vi "calculate image sharpness.vi"(8 "error in (no error)":errorcluster, 9 "Sharpness measure":T1, 11 "Autofocus in":refnum<class "Autofocus.lvclass">) -> (0 "error out":errorcluster, 2 "sharpness out":dbl, 3 "Autofocus out":refnum<class "Autofocus.lvclass">)   [LabVIEW 2012, in "Autofocus.lvclass"]
uses:
  Autofocus.lvclass
  Sharpness Measure.ctl
  Autofocus.lvclass/Autofocus.ctl
  search direction.ctl
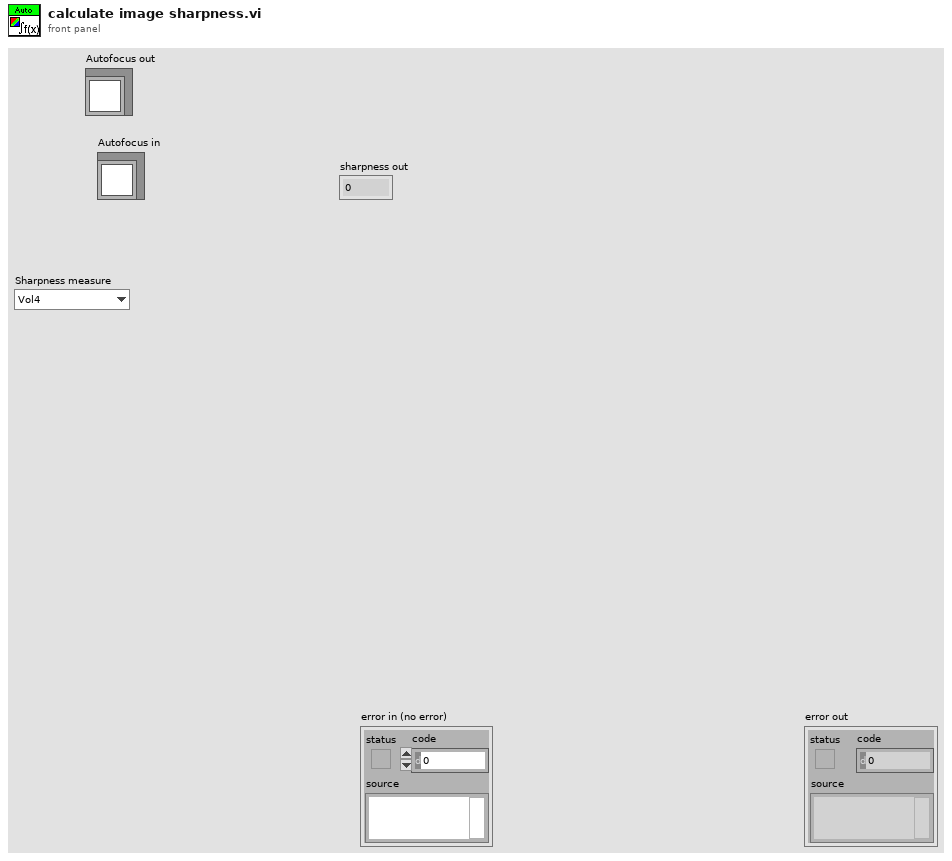
[diagram p1: front panel]
types:
  T1 = typedef "Autofocus.lvclass/Sharpness Measure.ctl" = enum16{"Vol4", "Gradient Square"}
  T2 = typedef "Autofocus.lvclass/search direction.ctl" = enum16{"going uphill", "going downhill", "idle"}
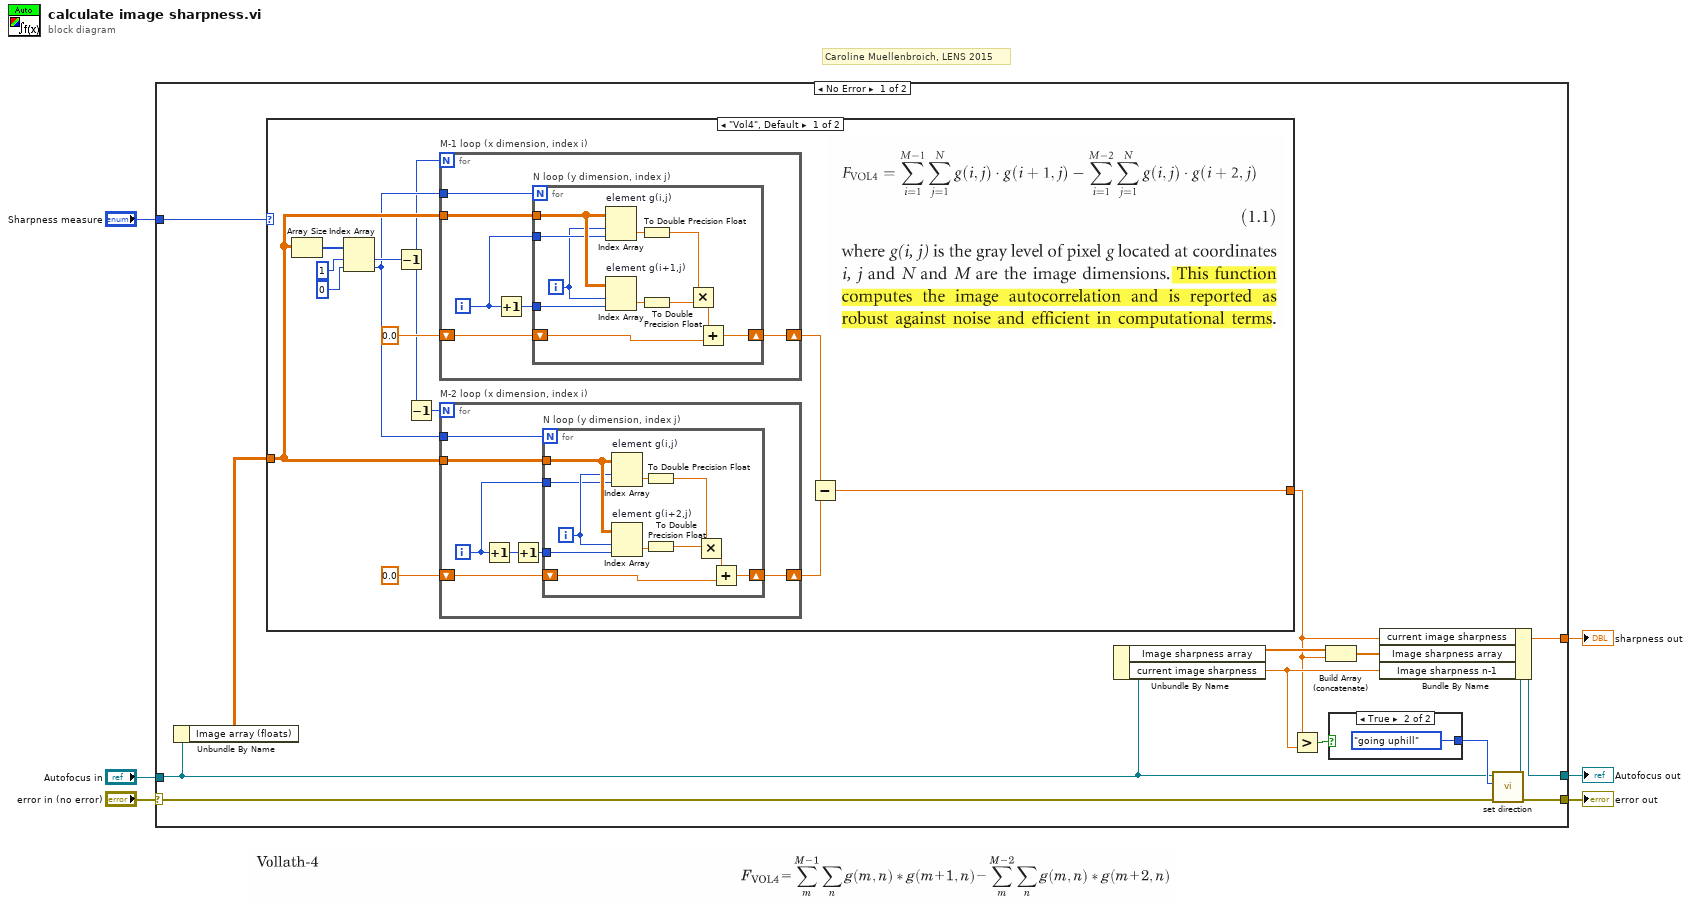
[diagram p0: block diagram]
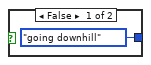
[diagram p2: hidden frame]
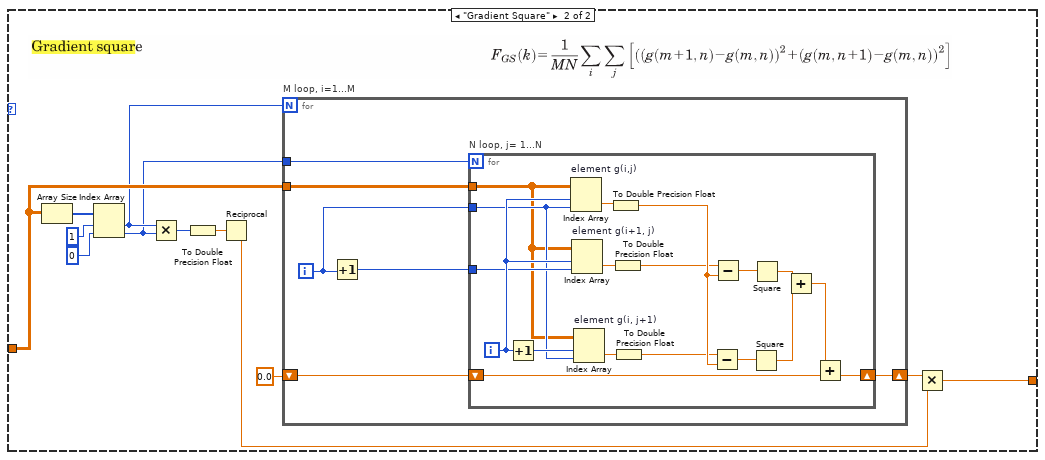
[diagram p3: hidden frame]
diagram:
  # "Caroline Muellenbroich, LENS 2015"
  n1 = case shown="No Error" "error in (no error)" {
    selector: "error in (no error)" -> [w10 w107]
    tunnel: [w15 w107] -> w5
    tunnel: [w19 w106] -> w3
    tunnel: "Autofocus in" -> [w8 w106]
    tunnel: [w11 _] -> w2
    tunnel: "Sharpness measure" -> [w18 _]
    frame No Error {
      n2 = Unbundle By Name(w8) -> ("Image array (floats)"=w7:dbl[][])
      n3 = case shown="\"Vol4\", Default" w18 {
        tunnel: w7 -> [w29 w78]
        tunnel: [w23 w73] -> w11
        frame "Vol4", Default {
          n4 = Array Size(array=w29) -> (size(s)=w34:i32[])
          n5 = Index Array(array=w34, index #1=1 ("index"), index #2=0 ("index")) -> (element #1=w30:i32, element #2=w28:i32)
          n6 = Decrement(x=w30) -> (x-1=w22:i32)
          n7 = Decrement(x=w22) -> (x-1=w31:i32)
          n8 = for "M-1 loop (x dimension, index i)" {
            N: w22 -> [_]
            tunnel: w29 -> [w58]
            tunnel: w28 -> [w57]
            shift-right: [w54] -> w27
            shift-left: 0.0 -> [w53]
            i -> [w56]
            n9 = Increment(x=w56) -> (x+1=w55:i32)
            n10 = for "N loop (y dimension, index j)" {
              N: w57 -> [_]
              tunnel: w58 -> [w68]
              shift-right: [w61] -> w54
              shift-left: w53 -> [w69]
              tunnel: w56 -> [w66]
              tunnel: w55 -> [w64]
              i -> [w65]
              n11 = Index Array "element g(i,j)"(array=w68, index (row)=w65, index (col)=w66) -> (element=w63:dbl)
              n12 = Index Array "element g(i+1,j)"(array=w68, index (row)=w65, index (col)=w64) -> (element=w62:dbl)
              n13 = To Double Precision Float(number=w63) -> (double precision float=w59:dbl)
              n14 = To Double Precision Float(number=w62) -> (double precision float=w60:dbl)
              n15 = Multiply(x=w59, y=w60) -> (x*y=w67:dbl)
              n16 = Add(x=w67, y=w69) -> (x+y=w61:dbl)
            }
          }
          n17 = for "M-2 loop (x dimension, index i)" {
            N: w31 -> [_]
            tunnel: w29 -> [w40]
            tunnel: w28 -> [w41]
            shift-right: [w36] -> w26
            shift-left: 0.0 -> [w35]
            i -> [w39]
            n18 = Increment(x=w39) -> (x+1=w38:i32)
            n19 = Increment(x=w38) -> (x+1=w37:i32)
            n20 = for "N loop (y dimension, index j)" {
              N: w41 -> [_]
              tunnel: w40 -> [w49]
              tunnel: w39 -> [w47]
              tunnel: w37 -> [w46]
              shift-right: [w45] -> w36
              shift-left: w35 -> [w44]
              i -> [w48]
              n21 = Index Array "element g(i,j)"(array=w49, index (row)=w48, index (col)=w47) -> (element=w51:dbl)
              n22 = Index Array "element g(i+2,j)"(array=w49, index (row)=w48, index (col)=w46) -> (element=w52:dbl)
              n23 = To Double Precision Float(number=w51) -> (double precision float=w42:dbl)
              n24 = To Double Precision Float(number=w52) -> (double precision float=w43:dbl)
              n25 = Multiply(x=w42, y=w43) -> (x*y=w50:dbl)
              n26 = Add(x=w50, y=w44) -> (x+y=w45:dbl)
            }
          }
          n27 = Subtract(x=w27, y=w26) -> (x-y=w23:dbl)
        }
        frame "Gradient Square" {
          n28 = Array Size(array=w78) -> (size(s)=w81:i32[])
          n29 = Index Array(array=w81, index #1=1 ("index"), index #2=0 ("index")) -> (element #1=w71:i32, element #2=w70:i32)
          n30 = Multiply(x=w71, y=w70) -> (x*y=w77:i32)
          n31 = To Double Precision Float(number=w77) -> (double precision float=w76:dbl)
          n32 = Reciprocal(x=w76) -> (1/x=w72:dbl)
          n33 = for "M loop, i=1...M" {
            N: w71 -> [_]
            tunnel: w78 -> [w87]
            tunnel: w70 -> [w86]
            shift-right: [w83] -> w74
            shift-left: 0.0 -> [w82]
            i -> [w85]
            n34 = Increment(x=w85) -> (x+1=w84:i32)
            n35 = for "N loop, j= 1...N" {
              N: w86 -> [_]
              tunnel: w87 -> [w101]
              tunnel: w85 -> [w102]
              tunnel: w84 -> [w104]
              shift-right: [w91] -> w83
              shift-left: w82 -> [w93]
              i -> [w105]
              n36 = Increment(x=w105) -> (x+1=w103:i32)
              n37 = Index Array "element g(i,j)"(array=w101, index (row)=w105, index (col)=w102) -> (element=w96:dbl)
              n38 = Index Array "element g(i+1, j)"(array=w101, index (row)=w105, index (col)=w104) -> (element=w100:dbl)
              n39 = Index Array "element g(i, j+1)"(array=w101, index (row)=w103, index (col)=w102) -> (element=w97:dbl)
              n40 = To Double Precision Float(number=w96) -> (double precision float=w90:dbl)
              n41 = To Double Precision Float(number=w100) -> (double precision float=w89:dbl)
              n42 = To Double Precision Float(number=w97) -> (double precision float=w88:dbl)
              n43 = Subtract(x=w88, y=w90) -> (x-y=w98:dbl)
              n44 = Subtract(x=w89, y=w90) -> (x-y=w99:dbl)
              n45 = Square(x=w98) -> (x^2=w94:dbl)
              n46 = Square(x=w99) -> (x^2=w95:dbl)
              n47 = Add(x=w95, y=w94) -> (x+y=w92:dbl)
              n48 = Add(x=w92, y=w93) -> (x+y=w91:dbl)
            }
          }
          n49 = Multiply(x=w74, y=w72) -> (x*y=w73:dbl)
        }
      }
      n50 = Unbundle By Name(w8) -> ("Image sharpness array"=w17:dbl[], "current image sharpness"=w13:dbl)
      n51 = Greater?(x=w11, y=w13) -> (0:w9:bool)
      n52 = Build Array (concatenate)(w17, w11) -> (w12:dbl[])
      n53 = case shown="True" w9 {
        tunnel: [search_direction."going downhill" ("search direction") search_direction."going uphill" ("search direction")] -> w16
        frame False {
        }
        frame True {
        }
      }
      n54 = call-dynamic "set direction.vi"("error in (no error)"=w10, "search direction"=w16, "Autofocus in"=w8) -> ("error out"=w15:errorcluster, "Autofocus out"=w14:refnum<class "Autofocus.lvclass">)  [unwired: 7 in]
      n55 = Bundle By Name(cluster=w14, "current image sharpness"=w11, "Image sharpness array"=w12, "Image sharpness n-1"=w13) -> (w19:refnum<class "Autofocus.lvclass">)
    }
    frame Error {
    }
  }
  "error out" <- w5
  "Autofocus out" <- w3
  "sharpness out" <- w2
